vi "specialUrlEncode.vi"(11 "str":string) -> (3 "UrlEncode":string)   [LabVIEW 2016, in "数据传输系统-04.lvlib" / "update.lvlib" / "http client.lvclass"]
uses:
  http client.lvclass
  System.Web
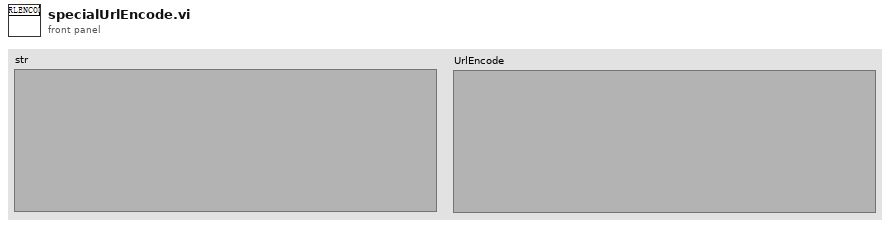
[diagram p1: front panel]
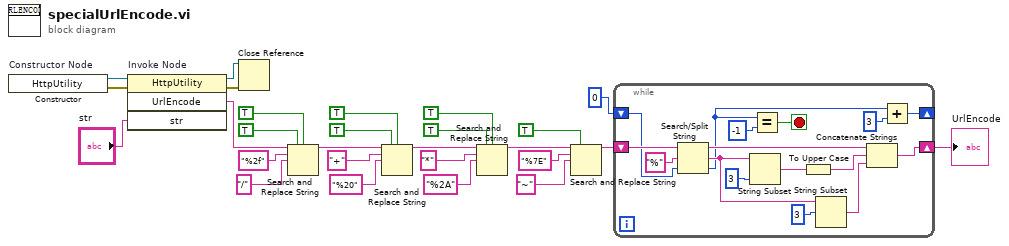
[diagram p0: block diagram]
diagram:
  n1 = constructor on="Constructor Node" class="HttpUtility"() -> (reference out=w27:refnum<k24>, error out=w26:errorcluster)  [unwired: 3 in, 1 out]
  n2 = invoke on="Invoke Node" class="HttpUtility" method="UrlEncode"(reference=w27, error in=w26, "str"="str") -> (reference out=w24:refnum<k24>, error out=w25:errorcluster, "UrlEncode"=w2:string)  [unwired: 1 in, 1 out]
  n3 = Close Reference(reference=w24, error in (no error)=w25) -> ()  [unwired: 1 out]
  n4 = Search and Replace String(replace all?=TRUE ("替换全部？(F)"), case sensitive?=TRUE ("忽略大小写？(F)"), input string=w2, search string="%2f" ("替换字符串(\"\")"), replace string="/" ("搜索字符串")) -> (result string=w1:string)  [unwired: 3 in, 3 out]
  n5 = Search and Replace String(replace all?=TRUE ("替换全部？(F)"), case sensitive?=TRUE ("忽略大小写？(F)"), input string=w1, search string="+" ("搜索字符串"), replace string="%20" ("替换字符串(\"\")")) -> (result string=w9:string)  [unwired: 3 in, 3 out]
  n6 = Search and Replace String(replace all?=TRUE ("替换全部？(F)"), case sensitive?=TRUE ("忽略大小写？(F)"), input string=w9, search string="*" ("搜索字符串"), replace string="%2A" ("替换字符串(\"\")")) -> (result string=w18:string)  [unwired: 3 in, 3 out]
  n7 = Search and Replace String(replace all?=TRUE ("替换全部？(F)"), input string=w18, search string="%7E" ("搜索字符串"), replace string="~" ("替换字符串(\"\")")) -> (result string=w12:string)  [unwired: 4 in, 3 out]
  n8 = while {
    shift-right: [w33] -> w13
    shift-left: w12 -> [w43]
    shift-right: [w39] -> _
    shift-left: 0 -> [w41]
    stop <- w30 stop-if-true
    n9 = Search/Split String(string=w43, search string/char (-)="%" ("搜索字符串/字符(-)"), offset (0)=w41) -> (substring before match=w35:string, match + rest of string=w37:string, offset of match=w32:i32)
    n10 = String Subset(string=w37, length (rest)=3 ("长度（剩余）")) -> (substring=w29:string)  [unwired: 1 in]
    n11 = Equal?(x=w32, y=-1) -> (x = y?=w30:bool)
    n12 = To Upper Case(1:w29) -> (0:w28:string)
    n13 = String Subset(string=w37, offset (0)=3 ("偏移量(0)")) -> (substring=w34:string)  [unwired: 1 in]
    n14 = Concatenate Strings(w35, w28, w34) -> (w33:string)
    n15 = Add(x=w32, y=3) -> (x+y=w39:i32)
  }
  "UrlEncode" <- w13
